vi "Draw BotPose Field.vi"(10 "Botpose":cluster{dbl, dbl}[](array[cluster]), 11 "Bordeaux":cluster{dbl, dbl}[](array[cluster])) -> ()   [LabVIEW 2025]
uses:
  <vilib>/picture/cartesn2.llb/XY Plot Type.ctl
panel:
  out "size(s)":i32
  in  "index":i32
  in  "Mode":T1(ring)
  in  "top left point(0, 0)":cluster{"x":i16, "y":i16}={"x"=-11, "y"=0}
  in  "[sized scatter plot cosmetics]":T2={"min size"=1, "max size"=5, "maps to max size"=5, "color array"=[16776960, 65280, 16711680, 255]}
  in  "XY plot cosmetics":T4={"plot color"=16776960, "XY plot type"=enum."circles", "baseline"=0.0} {"baseline" format="%0.2f"}
  in  "cartesian grid cosmetics":T5={"line color"=6710886, "text color"=13421772, "tick length(3)"=3, "crossing axes"=TRUE, "visible grid?"=FALSE}
  in  "cartesian axis attributes":T6={"x minimum"=0.0, "x maximum"=8.05, "x log?"=FALSE, "x precision"=1, "x format"=enum."Decimal", "y minimum"=0.0, "y maximum"=17.55, "y log?"=FALSE, "y precision"=1, "y format"=enum."Decimal"} {"x minimum" format="%0.2f"; "x maximum" format="%0.2f"; "y minimum" format="%0.2f"; "y maximum" format="%0.2f"}
  out "new picture":picture
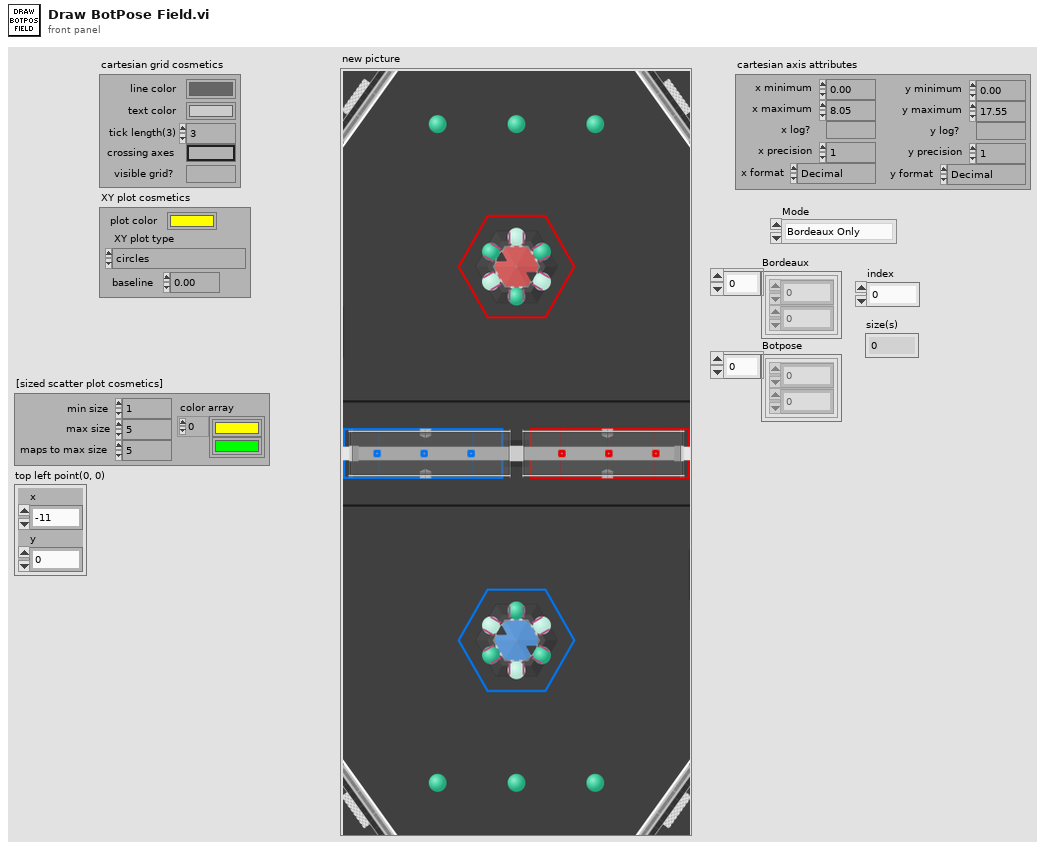
[diagram p1: front panel]
types:
  T1 = enum16{"Bordeaux Only", "BotPose Only", "One Point of Each"}
  T2 = cluster{"min size":i16, "max size":i16, "maps to max size":i16, "color array":u32[]}
  T3 = typedef "XY Plot Type.ctl" = enum16{"points", "squares", "circles", "connected points", "connected squares", "connected circles", "comb plot", "sized scatter plot", "sized-colored scatter plot", "min-max lines"}
  T4 = cluster{"plot color":u32, "XY plot type":T3, "baseline":dbl}
  T5 = cluster{"line color":u32, "text color":u32, "tick length(3)":i16, "crossing axes":bool, "visible grid?":bool}
  T6 = cluster{"x minimum":dbl, "x maximum":dbl, "x log?":bool, "x precision":u8, "x format":enum8{"Decimal", "Scientific", "Engineering", "Binary", "Octal", "Hex"}, "y minimum":dbl, "y maximum":dbl, "y log?":bool, "y precision":u8, "y format":enum8{"Decimal", "Scientific", "Engineering", "Binary", "Octal", "Hex"}}
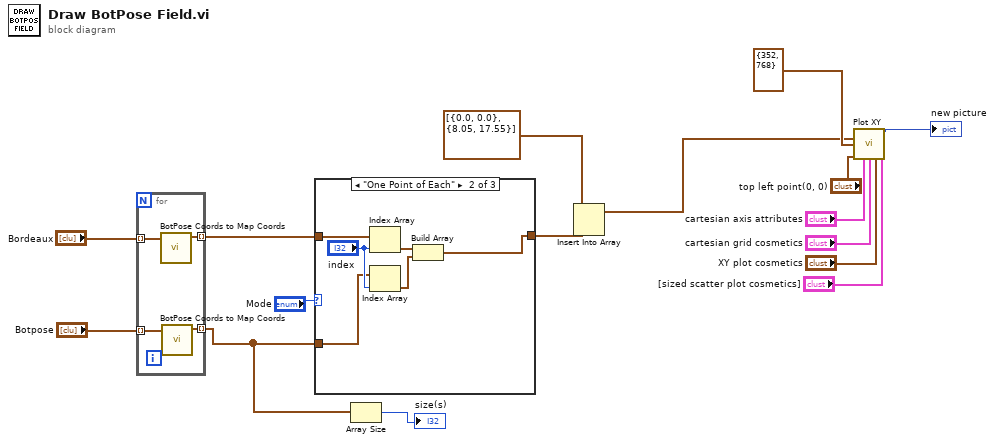
[diagram p0: block diagram]
diagram:
  n1 = for {
    tunnel: "Bordeaux" -> [w20] mode=indexing
    tunnel: "Botpose" -> [w19] mode=indexing
    tunnel: [w18] -> w5 mode=indexing
    tunnel: [w17] -> w4 mode=indexing
    n2 = call "BotPose Coords to Map Coords.vi"("Point In"=w20) -> ("Point Out"=w18:cluster{dbl, dbl})  [unwired: 10 in]
    n3 = call "BotPose Coords to Map Coords.vi"("Point In"=w19) -> ("Point Out"=w17:cluster{dbl, dbl})  [unwired: 10 in]
  }
  n4 = case shown="\"One Point of Each\"" "Mode" {
    tunnel: [w21 w22 w28] -> w3
    tunnel: w5 -> [w21 w26 _]
    tunnel: w4 -> [_ w25 w28]
    frame "Bordeaux Only", Default {
    }
    frame "One Point of Each" {
      n5 = Index Array(array=w26, index="index") -> (element=w24:cluster{dbl, dbl})
      n6 = Index Array(array=w25, index="index") -> (element=w23:cluster{dbl, dbl})
      n7 = Build Array(w24, w23) -> (w22:cluster{dbl, dbl}[])
    }
    frame "BotPose Only" {
    }
  }
  n8 = Array Size(array=w4) -> (size(s)=→"size(s)":i32)
  n9 = Insert Into Array(array=cluster{dbl, dbl}[] [{0.0, 0.0}, {8.05, 17.55}], new element=w3) -> (w1:cluster{dbl, dbl}[])  [unwired: 1 in]
  n10 = call <vilib>:"Plot XY.vi"("data"=w1, "dimensions (w,h)"=cluster{"width":i16, "height":i16} {"width"=352, "height"=768}, "top left point(0, 0)"="top left point(0, 0)", "cartesian axis attributes"="cartesian axis attributes", "cartesian grid cosmetics"="cartesian grid cosmetics", "XY plot cosmetics"="XY plot cosmetics", "[sized scatter plot cosmetics]"="[sized scatter plot cosmetics]") -> ("new picture"=→"new picture":picture)  [unwired: 8 in]
